vi "PipBoy_Main.vi"() -> ()   [LabVIEW 2014]
uses:
  ctls/PipBoy_LabVIEWEvent.ctl
  ctls/PipBoy_DetectionType.ctl
  <vilib>/ErrorRing/Error Ring.xnode
  modules/support/Message Queue/Message Queue.lvlib
  modules/support/User Event - Stop/User Event - Stop.lvlib
panel:
  in  "Command":string="Add"
  out "PipBoy":string
  in  "Cmd":bool
  in  "Stop":bool
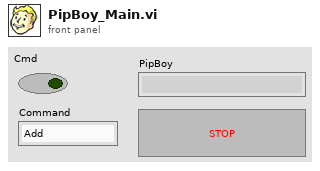
[diagram p1: front panel]
types:
  T1 = enum32{"Invalid", "Standard", "Closed", "Hidden", "Minimized", "Maximized"}
  T2 = typedef "PipBoy_PipBoyData.ctl" = cluster{"ProcComm":T3, "FileConf":T5, "PicComm":T6, "GnlPrms":T7, "Pages":T8}
  T3 = typedef "PipBoy_ProcComm.ctl" = cluster{"NotifyIconRef":refnum<k24>, "UE-Stop":refnum<user-event>, "UE-PipboyCommand":refnum<user-event>, "UE-UpdateData":refnum<user-event>, "MsgQ":T4}
  T4 = typedef "Message Queue.lvlib/All Message Queues.ctl" = cluster{"UI":refnum<queue>, "PipCom":refnum<queue>}
  T5 = typedef "PipBoy_FileConf.ctl" = cluster{"VisaPic32":refnum<visa-resource-name>, "LabVIEWPorts":u16[], "DEBUG":bool, "IconFilePath":path, "IconsNbByPage":i32}
  T6 = typedef "PipBoy_PicComm.ctl" = cluster{"PicInit?":bool}
  T7 = typedef "PipBoy_GeneralParams.ctl" = cluster{"IconPath":path, "LabVIEWs":refnum<vi>[], "ActiveLabVIEW":i32, "OpenedPorts":u16[], "ContextMenu":string[][]}
  T8 = typedef "PipBoy_Pages.ctl" = cluster{"PageNum":i32, "Functions":string[]}
  T9 = cluster{"UE-Stop":refnum<event-registration>, "UE-NotifyMenu":refnum<event-registration>, "UE-PipBoyCmd":refnum<event-registration>, "UE-UpdateData":refnum<event-registration>}
  T10 = typedef "PipBoy_LabVIEWEvent.ctl" = cluster{"DetecType":T11, "LvVersion":string, "Index":i32}
  T11 = typedef "PipBoy_DetectionType.ctl" = enum16{"Detected", "Lost"}
  T12 = typedef "NotifyIcon Event Data.ctl" = cluster{"NotifyIcon Event":T13, "Data String":string}
  T13 = typedef "NotifyIcon Events.ctl" = enum16{"BalloonTipClicked", "BalloonTipClosed", "BalloonTipShown", "Click", "Disposed", "DoubleClick", "MouseClick", "MouseDoubleClick", "MouseDown", "MouseMove", "MouseUp", "MenuItemClick", "MenuItemSelect"}
  T14 = enum32{"invalid app kind", "Development System", "Run Time System", "Student Edition", "Embedded LabVIEW", "Evaluation", "Custom"}
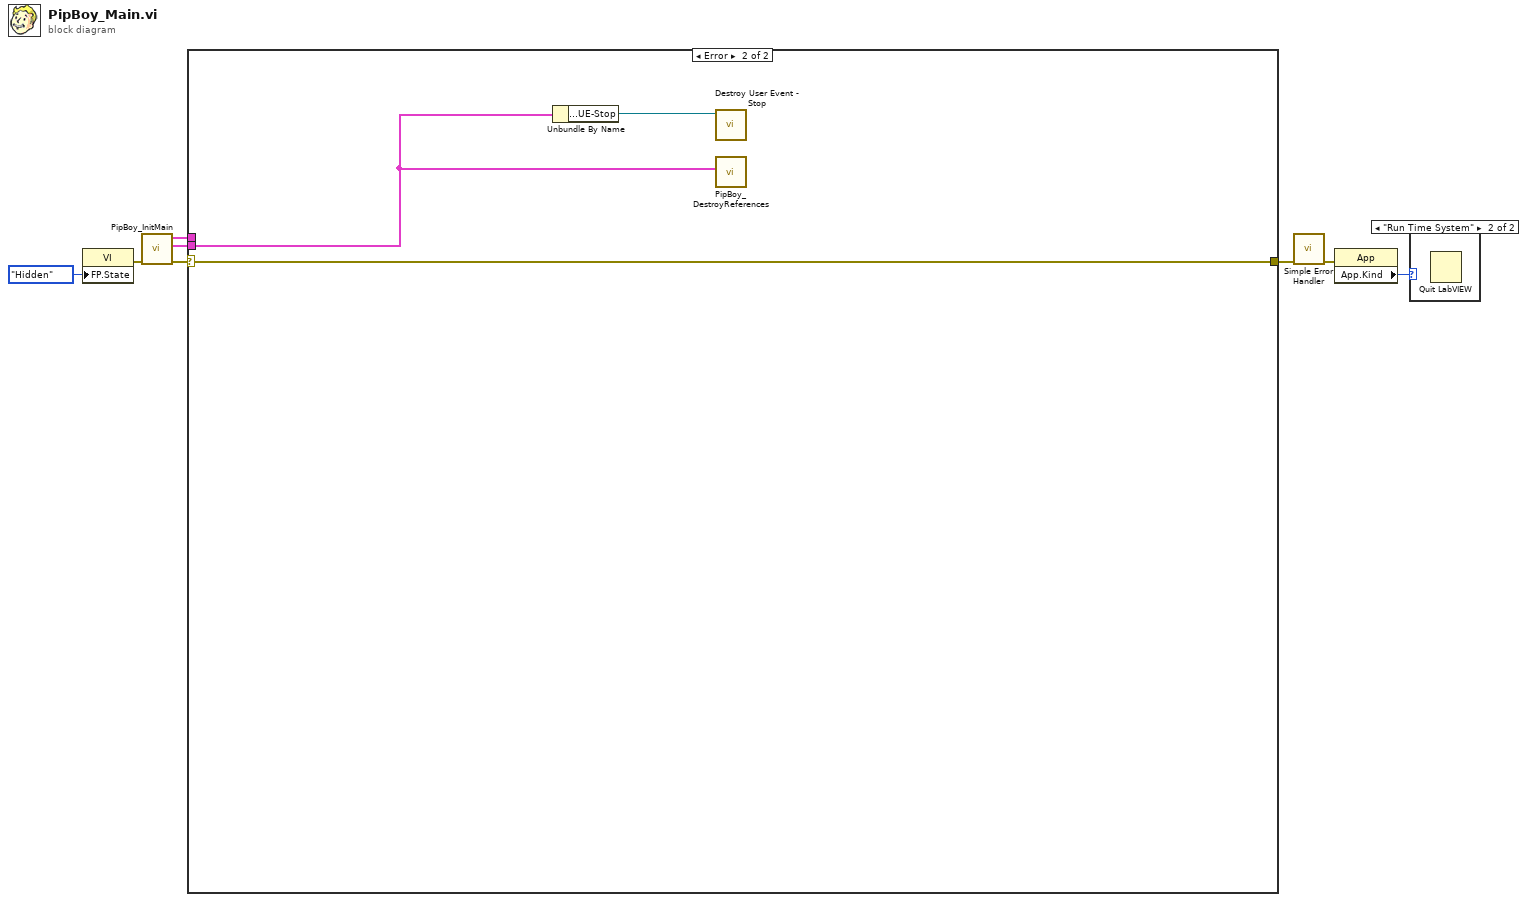
[diagram p0: block diagram]
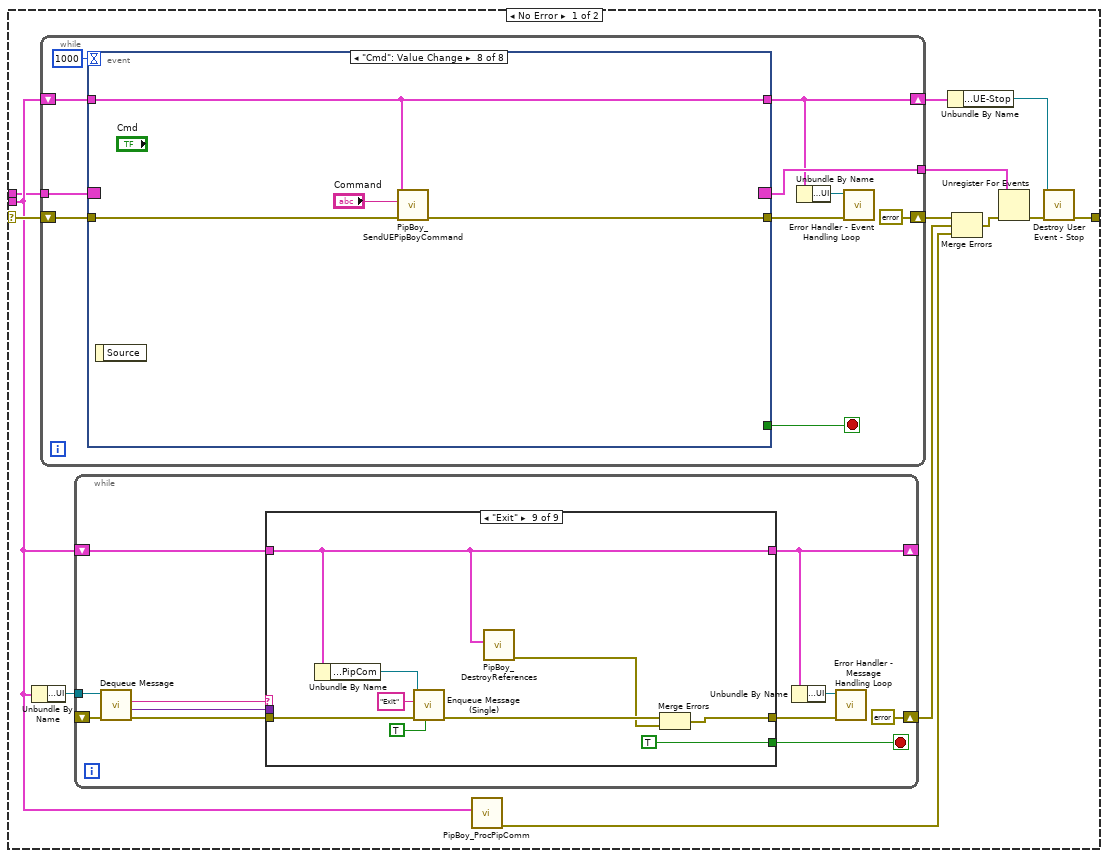
[diagram p2: hidden frame]
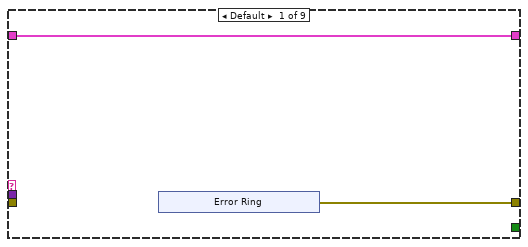
[diagram p3: hidden frame]
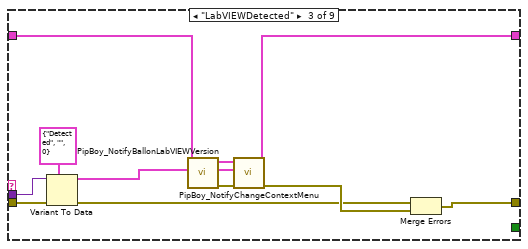
[diagram p5: hidden frame]
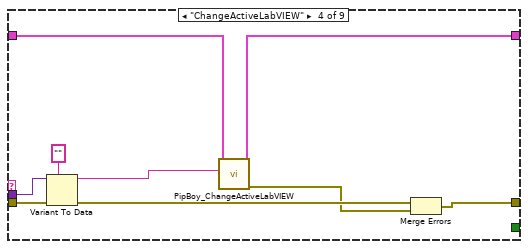
[diagram p6: hidden frame]
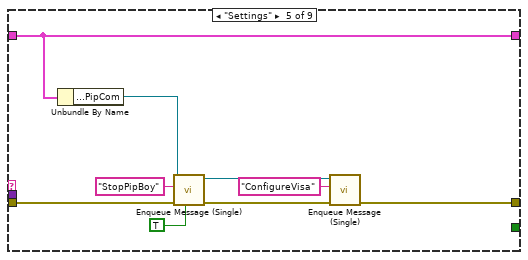
[diagram p7: hidden frame]
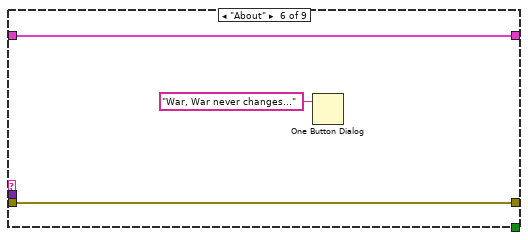
[diagram p8: hidden frame]
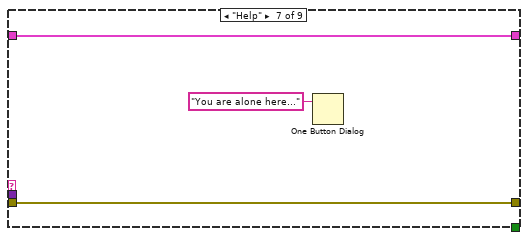
[diagram p9: hidden frame]
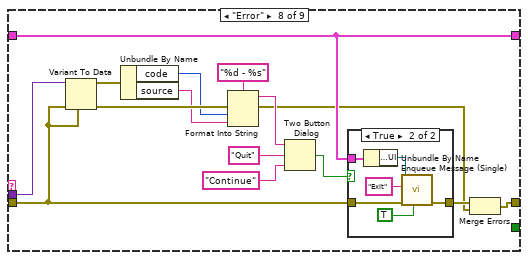
[diagram p10: hidden frame]
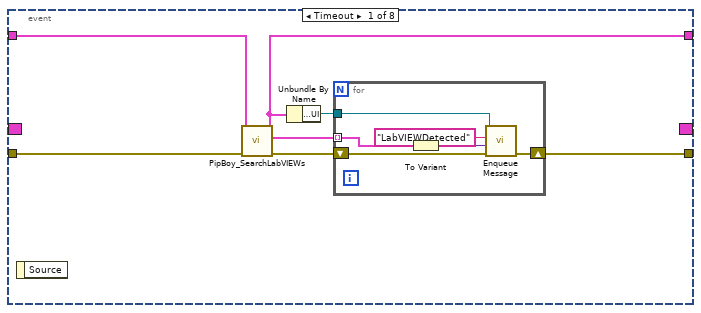
[diagram p12: hidden frame]
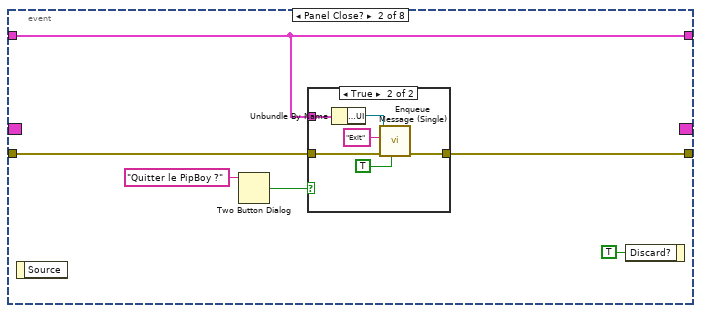
[diagram p13: hidden frame]
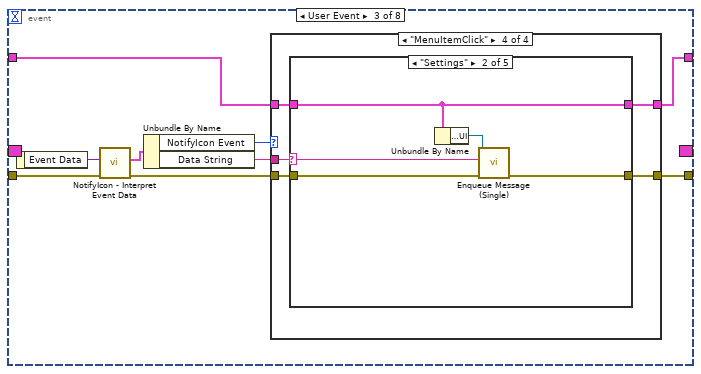
[diagram p15: hidden frame]
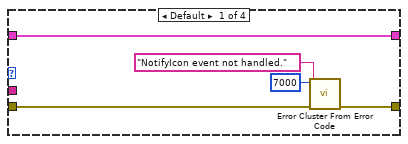
[diagram p16: hidden frame]
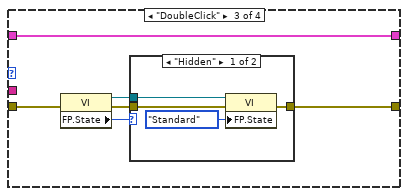
[diagram p18: hidden frame]
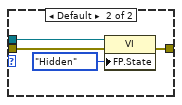
[diagram p19: hidden frame]
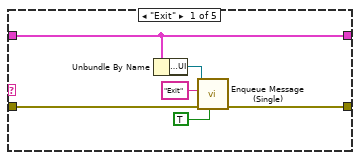
[diagram p20: hidden frame]
diagram:
  n1 = property class="VI"("FP.State"=T1."Hidden" ("Front Panel Window:State")) -> (error out=w3:errorcluster)  [unwired: 2 in, 1 out]
  n2 = call "PipBoy_InitMain.vi"("error in (no error)"=w3) -> ("error out"=w5:errorcluster, "PipBoyData"=w6:T2, "DynamicUE"=w1:T9)  [unwired: 8 in]
  n3 = case shown="Error" w5 {
    selector: w5 -> [w11 w286]
    tunnel: [w16 w286] -> w7
    tunnel: w6 -> [w10 w285]
    tunnel: w1 -> [w9 _]
    frame No Error {
      n4 = Unbundle By Name(w10) -> ("ProcComm.MsgQ.UI"=w18:refnum<queue>)
      n5 = while {
        tunnel: [w115] -> w19
        shift-right: [w112] -> w13
        shift-left: w10 -> [w113]
        shift-right: [errorcluster {"status"=FALSE, "code"=0, "source"=""} ("error IO")] -> w21
        shift-left: w11 -> [w118]
        tunnel: w9 -> [w109]
        stop <- w117 stop-if-true
        n6 = event shown="[7] \"Cmd\": Value Change" {
          selector: w109 -> [_ _ _ _ _ _ _ _]
          dyn-events: [_ _ _ _ _ _ _ _] -> w115
          timeout: 1000 -> [_ _ _ _ _ _ _ _]
          tunnel: w118 -> [w125 w135 w153 w230 w243 w264 w279 w282]
          tunnel: [_ _ _ TRUE ("Discard?") _ _ _ _] -> w117
          tunnel: [w122 w134 w148 w230 w242 w263 w276 w281] -> w116
          tunnel: w113 -> [w124 w132 w146 w229 w234 w260 w275 w283]
          tunnel: [w119 w132 w145 w229 w233 w259 w275 w283] -> w112
          event Timeout {
            n7 = event-data() -> ()  [unwired: 1 in, 1 out]
            n8 = call "PipBoy_SearchLabVIEWs.vi"("error in (no error)"=w125, "PipBoyDataIn"=w124) -> ("error out"=w123:errorcluster, "LabVIEWEvents"=w120:T10[], "PipBoyDataOut"=w119:T2)  [unwired: 7 in]
            n9 = Unbundle By Name(w119) -> ("ProcComm.MsgQ.UI"=w121:refnum<queue>)
            n10 = for {
              shift-right: [w129] -> w122
              shift-left: w123 -> [w130]
              tunnel: w121 -> [w126]
              tunnel: w120 -> [w128] mode=indexing
              n11 = To Variant(anything=w128) -> (Variant=w127:variant)
              n12 = call-poly "Enqueue Message.vi"("error in (no error)"=w130, "Message Data"=w127, "Message"="LabVIEWDetected", "Message Queue"=w126) -> ("error out"=w129:errorcluster)  [unwired: 6 in, 1 out]
            }
          }
          event Panel Close? {
            n13 = event-data() -> ()  [unwired: 1 in, 1 out]
            n14 = Two Button Dialog(message="Quitter le PipBoy ?") -> (T button?=w133:bool)  [unwired: 2 in]
            n15 = case shown="True" w133 {
              tunnel: w135 -> [w138 w142]
              tunnel: [w138 w141] -> w134
              tunnel: w132 -> [_ w140]
              frame False {
              }
              frame True {
                n16 = Unbundle By Name(w140) -> ("ProcComm.MsgQ.UI"=w139:refnum<queue>)
                n17 = call "Enqueue Message (Single).vi"("Priority Message? (F)"=TRUE, "error in (no error)"=w142, "Message"="Exit", "Message Queue"=w139) -> ("error out"=w141:errorcluster)  [unwired: 6 in, 1 out]
              }
            }
            n18 = event-data("Discard?"=TRUE) -> ()  [unwired: 1 in, 1 out]
          }
          event User Event {
            n19 = event-data() -> ("Event Data"=w152:variant)  [unwired: 1 in]
            n20 = call <userlib>:"NotifyIcon - Interpret Event Data.vi"("error in"=w153, "NotifyIcon Event Data"=w152) -> ("error out"=w149:errorcluster, "NotifyIcon Event Data"=w151:T12)  [unwired: 8 in]
            n21 = Unbundle By Name(w151) -> ("NotifyIcon Event"=w150:T13, "Data String"=w147:string)
            n22 = case shown="\"MenuItemClick\"" w150 {
              tunnel: w149 -> [w157 w160 w164 w178]
              tunnel: [w158 w160 w162 w177] -> w148
              tunnel: w147 -> [_ _ _ w179]
              tunnel: w146 -> [w154 w159 w161 w176]
              tunnel: [w154 w159 w161 w175] -> w145
              frame Default {
                n23 = call <vilib>:"Error Cluster From Error Code.vi"("error in (no error)"=w157, "error message (\"\")"="NotifyIcon event not handled." ("error message (\"\")"), "error code (0)"=7000) -> ("error out"=w158:errorcluster)  [unwired: 6 in]
              }
              frame "BalloonTipClicked" {
              }
              frame "DoubleClick" {
                n24 = property class="VI"(error in=w164) -> (reference out=w165:refnum<vi>, error out=w163:errorcluster, "FP.State"=w166:T1)  [unwired: 1 in]
                n25 = case shown="\"Hidden\"" w166 {
                  tunnel: w165 -> [w168 w171]
                  tunnel: w163 -> [w170 w173]
                  tunnel: [w169 w172] -> w162
                  frame "Hidden" {
                    n26 = property class="VI"(reference=w168, error in=w170, "FP.State"=T1."Standard" ("Front Panel Window:State")) -> (error out=w169:errorcluster)  [unwired: 1 out]
                  }
                  frame Default {
                    n27 = property class="VI"(reference=w171, error in=w173, "FP.State"=T1."Hidden" ("Front Panel Window:State")) -> (error out=w172:errorcluster)  [unwired: 1 out]
                  }
                }
              }
              frame "MenuItemClick" {
                n28 = case shown="\"Settings\"" w179 {
                  selector: w179 -> [_ w187 w192 w197 w213]
                  tunnel: w178 -> [w183 w189 w194 w199 w204]
                  tunnel: [w182 w188 w193 w198 w203] -> w177
                  tunnel: w176 -> [w180 w186 w191 w196 w202]
                  tunnel: [w180 w186 w191 w196 w201] -> w175
                  frame "Exit" {
                    n29 = Unbundle By Name(w180) -> ("ProcComm.MsgQ.UI"=w181:refnum<queue>)
                    n30 = call "Enqueue Message (Single).vi"("Priority Message? (F)"=TRUE, "error in (no error)"=w183, "Message"="Exit", "Message Queue"=w181) -> ("error out"=w182:errorcluster)  [unwired: 6 in, 1 out]
                  }
                  frame "Settings" {
                    n31 = Unbundle By Name(w186) -> ("ProcComm.MsgQ.UI"=w190:refnum<queue>)
                    n32 = call "Enqueue Message (Single).vi"("error in (no error)"=w189, "Message"=w187, "Message Queue"=w190) -> ("error out"=w188:errorcluster)  [unwired: 7 in, 1 out]
                  }
                  frame "About" {
                    n33 = Unbundle By Name(w191) -> ("ProcComm.MsgQ.UI"=w195:refnum<queue>)
                    n34 = call "Enqueue Message (Single).vi"("error in (no error)"=w194, "Message"=w192, "Message Queue"=w195) -> ("error out"=w193:errorcluster)  [unwired: 7 in, 1 out]
                  }
                  frame "Help" {
                    n35 = Unbundle By Name(w196) -> ("ProcComm.MsgQ.UI"=w200:refnum<queue>)
                    n36 = call "Enqueue Message (Single).vi"("error in (no error)"=w199, "Message"=w197, "Message Queue"=w200) -> ("error out"=w198:errorcluster)  [unwired: 7 in, 1 out]
                  }
                  frame Default {
                    n37 = Spreadsheet String To Array(delimiter (Tab)="\\", format string="", spreadsheet string=w213, array type (2D Dbl)=string[] []) -> (array=w211:string[])
                    n38 = Index Array(array=w211) -> (element #1=w209:string, element #2=w208:string)  [unwired: 2 in]
                    n39 = case shown="\"Active LabVIEW\"" w209 {
                      tunnel: w208 -> [_ w221 w224]
                      tunnel: "A town has been desolated..." -> [_ w219 _]
                      tunnel: "Barraux has been desolated..." -> [_ w218 _]
                      tunnel: w204 -> [w214 w216 w228]
                      tunnel: [w214 w216 w227] -> w203
                      tunnel: w202 -> [w215 w217 w226]
                      tunnel: [w215 w217 w225] -> w201
                      frame Default {
                      }
                      frame "Nuclear Strike" {
                        n40 = case shown="\"Random city\"" w221 {
                          tunnel: [w222 w223] -> w220
                          tunnel: w219 -> [w222 _]
                          tunnel: w218 -> [_ w223]
                          frame Default {
                          }
                          frame "Random city" {
                          }
                        }
                        n41 = One Button Dialog(message=w220) -> ()  [unwired: 1 in, 1 out]
                      }
                      frame "Active LabVIEW" {
                        n42 = call "PipBoy_ChangeActiveLabVIEW.vi"("error in (no error)"=w228, "LvVersion"=w224, "PipBoyDataIn"=w226) -> ("error out"=w227:errorcluster, "PipBoyDataOut"=w225:T2)  [unwired: 7 in]
                      }
                    }
                  }
                }
              }
            }
          }
          event User Event {
            n43 = event-data() -> ()  [unwired: 1 in, 1 out]
          }
          event User Event {
            n44 = event-data() -> ("Name"=w232:string)  [unwired: 1 in]
            "PipBoy" <- w232
            n45 = Spreadsheet String To Array(delimiter (Tab)="=", format string="", spreadsheet string=w232, array type (2D Dbl)=string[] []) -> (array=w238:string[])
            n46 = Index Array(array=w238) -> (element #1=w237:string, element #2=w236:string)  [unwired: 2 in]
            n47 = case shown="\"Icon\"" w237 {
              tunnel: [w246 w250 w253 w257] -> w242
              tunnel: w234 -> [w245 w247 w252 w256]
              tunnel: w243 -> [w246 w249 w254 w258]
              tunnel: w236 -> [_ w248 _ _]
              tunnel: [w245 w247 w251 w255] -> w233
              frame Default {
              }
              frame "Icon" {
                n48 = call "PipBoy_SendCommandToLabVIEW.vi"("error in (no error)"=w249, "Command"=w248, "PipBoyDataIn"=w247) -> ("error out"=w250:errorcluster)  [unwired: 8 in]
              }
              frame "Previous" {
                n49 = call "PipBoy_Cmd-Previous.vi"("error in (no error)"=w254, "DataIn"=w252) -> ("error out"=w253:errorcluster, "DataOut"=w251:T2)  [unwired: 8 in]
              }
              frame "Next" {
                n50 = call "PipBoy_Cmd-Next.vi"("error in (no error)"=w258, "DataIn"=w256) -> ("error out"=w257:errorcluster, "DataOut"=w255:T2)  [unwired: 8 in]
              }
            }
            n51 = Unbundle By Name(w234) -> ("FileConf.DEBUG"=w241:bool)
            n52 = case shown="True" w241 {
              tunnel: w232 -> [_ w244]
              frame False {
              }
              frame True {
                n53 = One Button Dialog(message=w244) -> ()  [unwired: 1 in, 1 out]
              }
            }
          }
          event User Event {
            n54 = event-data() -> ("Name"=w262:string, "Data"=w261:variant)  [unwired: 1 in]
            n55 = case shown="\"ContextMenu\"" w262 {
              tunnel: [w266 w270] -> w263
              tunnel: w264 -> [w266 w271]
              tunnel: w261 -> [_ w269]
              tunnel: [w265 w272] -> w259
              tunnel: w260 -> [w265 w273]
              frame Default {
              }
              frame "ContextMenu" {
                n56 = Variant To Data(error in=w271, type=string[][] [] ("GnlPrms.ContextMenu"), Variant=w269) -> (data=w267:string[][], error out=w270:errorcluster)
                n57 = Bundle By Name(cluster=w273, "GnlPrms.ContextMenu"=w267) -> (w272:T2)
              }
            }
          }
          event "Stop": Value Change {
            n58 = event-data() -> ()  [unwired: 1 in, 1 out]
            n59 = Unbundle By Name(w275) -> ("ProcComm.MsgQ.UI"=w274:refnum<queue>)
            n60 = call "Enqueue Message (Single).vi"("Priority Message? (F)"=TRUE, "error in (no error)"=w279, "Message"="Exit", "Message Queue"=w274) -> ("error out"=w276:errorcluster)  [unwired: 6 in, 1 out]
          }
          event "Cmd": Value Change {
            n61 = event-data() -> ()  [unwired: 1 in, 1 out]
            n62 = call "PipBoy_SendUEPipBoyCommand.vi"("error in (no error)"=w282, "Command"="Command", "PipBoyData"=w283) -> ("error out"=w281:errorcluster)  [unwired: 8 in]
          }
        }
        n63 = Unbundle By Name(w112) -> ("ProcComm.MsgQ.UI"=w114:refnum<queue>)
        n64 = call "Error Handler - Event Handling Loop.vi"("error in (no error)"=w116, "Message Queue"=w114) -> ()  [unwired: 8 in, 2 out]
      }
      n65 = while {
        tunnel: w18 -> [w24]
        shift-right: [errorcluster {"status"=FALSE, "code"=0, "source"=""} ("error IO")] -> w14
        shift-left: _ -> [w32]
        shift-right: [w25] -> _
        shift-left: w10 -> [w28]
        stop <- w27 stop-if-true
        n66 = call "Dequeue Message.vi"("error in (no error)"=w32, "Message Queue"=w24) -> ("error out"=w29:errorcluster, "Message Data"=w26:variant, "Message"=w31:string)  [unwired: 6 in, 1 out]
        n67 = case shown="\"Exit\"" w31 {
          tunnel: [w34 w40 w53 w62 w63 w73 w76 w83 w108] -> w30
          tunnel: w29 -> [_ w40 w47 w61 w70 w73 w76 w80 w104]
          tunnel: w28 -> [w33 w41 w52 w58 w69 w74 w77 w84 w100]
          tunnel: [w33 w41 w48 w57 w69 w74 w77 w84 w100] -> w25
          tunnel: [_ _ _ _ _ _ _ _ TRUE] -> w27
          tunnel: w26 -> [_ _ w44 w59 _ _ _ w92 _]
          frame Default {
            n68 = xnode "Error Ring"() -> ("error out"=w34:errorcluster)
          }
          frame "Initialize" {
          }
          frame "LabVIEWDetected" {
            n69 = Variant To Data(error in=w47, type=T10 {"DetecType"=enum."Detected", "LvVersion"="", "Index"=0} ("LabVIEWEvent"), Variant=w44) -> (data=w43:T10, error out=w46:errorcluster)
            n70 = call "PipBoy_NotifyBallonLabVIEWVersion.vi"("LabVIEWEventIn"=w43, "PipBoyDataIn"=w52) -> ("error out"=w51:errorcluster, "LabVIEWEventOut"=w42:T10, "PipBoyDataOut"=w49:T2)  [unwired: 7 in]
            n71 = call "PipBoy_NotifyChangeContextMenu.vi"("error in (no error)"=w51, "LabVIEWEvent"=w42, "PipBoyDataIn"=w49) -> ("error out"=w50:errorcluster, "PipBoyDataOut"=w48:T2)  [unwired: 7 in]
            n72 = Merge Errors(w46, w50) -> (w53:errorcluster)
          }
          frame "ChangeActiveLabVIEW" {
            n73 = Variant To Data(error in=w61, type="", Variant=w59) -> (data=w55:string, error out=w60:errorcluster)
            n74 = call "PipBoy_ChangeActiveLabVIEW.vi"("LvVersion"=w55, "PipBoyDataIn"=w58) -> ("error out"=w54:errorcluster, "PipBoyDataOut"=w57:T2)  [unwired: 8 in]
            n75 = Merge Errors(w60, w54) -> (w62:errorcluster)
          }
          frame "Settings" {
            n76 = Unbundle By Name(w69) -> ("ProcComm.MsgQ.PipCom"=w68:refnum<queue>)
            n77 = call "Enqueue Message (Single).vi"("Priority Message? (F)"=TRUE, "error in (no error)"=w70, "Message"="StopPipBoy", "Message Queue"=w68) -> ("error out"=w64:errorcluster, "dup Message Queue"=w67:refnum<queue>)  [unwired: 6 in]
            n78 = call "Enqueue Message (Single).vi"("error in (no error)"=w64, "Message"="ConfigureVisa", "Message Queue"=w67) -> ("error out"=w63:errorcluster)  [unwired: 7 in, 1 out]
          }
          frame "About" {
            n79 = One Button Dialog(message="War, War never changes...") -> ()  [unwired: 1 in, 1 out]
          }
          frame "Help" {
            n80 = One Button Dialog(message="You are alone here...") -> ()  [unwired: 1 in, 1 out]
          }
          frame "Error" {
            n81 = Variant To Data(error in=w80, type=w80, Variant=w92) -> (data=w91:errorcluster, error out=w90:errorcluster)
            n82 = Unbundle By Name(w91) -> ("code"=w89:i32, "source"=w87:string)
            n83 = Format Into String(format string="%d - %s", error in=w90, w89, w87) -> (resulting string=w86:string, error out=w81:errorcluster)  [unwired: 1 in]
            n84 = Two Button Dialog(message=w86, 1:"Continue" ("F button name (\"Cancel\")"), 2:"Quit" ("T button name (\"OK\")")) -> (T button?=w85:bool)
            n85 = case shown="True" w85 {
              tunnel: [w93 w97] -> w82
              tunnel: w80 -> [w93 w96]
              tunnel: w84 -> [_ w95]
              frame False {
              }
              frame True {
                n86 = Unbundle By Name(w95) -> ("ProcComm.MsgQ.UI"=w94:refnum<queue>)
                n87 = call "Enqueue Message (Single).vi"("Priority Message? (F)"=TRUE, "error in (no error)"=w96, "Message"="Exit", "Message Queue"=w94) -> ("error out"=w97:errorcluster)  [unwired: 6 in, 1 out]
              }
            }
            n88 = Merge Errors(w82, w81) -> (w83:errorcluster)
          }
          frame "Exit" {
            n89 = Unbundle By Name(w100) -> ("ProcComm.MsgQ.PipCom"=w103:refnum<queue>)
            n90 = call "Enqueue Message (Single).vi"("Priority Message? (F)"=TRUE, "error in (no error)"=w104, "Message"="Exit", "Message Queue"=w103) -> ("error out"=w102:errorcluster)  [unwired: 6 in, 1 out]
            n91 = call "PipBoy_DestroyReferences.vi"("PipBoyData"=w100) -> ("error out"=w101:errorcluster)  [unwired: 10 in]
            n92 = Merge Errors(w102, w101) -> (w108:errorcluster)
          }
        }
        n93 = Unbundle By Name(w25) -> ("ProcComm.MsgQ.UI"=w23:refnum<queue>)
        n94 = call "Error Handler - Message Handling Loop.vi"("error in (no error)"=w30, "Message Queue"=w23) -> ()  [unwired: 8 in, 2 out]
      }
      n95 = call "PipBoy_ProcPipComm.vi"("PipBoyData"=w10) -> ("error out"=w12:errorcluster)  [unwired: 10 in]
      n96 = Unbundle By Name(w13) -> ("ProcComm.UE-Stop"=w15:refnum<user-event>)
      n97 = Merge Errors(w21, w14, w12) -> (w20:errorcluster)
      n98 = Unregister For Events(event registration refnum=w19, error in=w20) -> (error out=w17:errorcluster)
      n99 = call "Destroy User Event - Stop.vi"("error in (no error)"=w17, "User Event - Stop"=w15) -> ("error out"=w16:errorcluster)  [unwired: 9 in]
    }
    frame Error {
      n100 = Unbundle By Name(w285) -> ("ProcComm.UE-Stop"=w284:refnum<user-event>)
      n101 = call "Destroy User Event - Stop.vi"("User Event - Stop"=w284) -> ()  [unwired: 10 in, 1 out]
      n102 = call "PipBoy_DestroyReferences.vi"("PipBoyData"=w285) -> ()  [unwired: 10 in, 1 out]
    }
  }
  n103 = call <vilib>:"Simple Error Handler.vi"("error in (no error)"=w7) -> ("error out"=w8:errorcluster)  [unwired: 4 in, 4 out]
  n104 = property class="App"(error in=w8) -> ("App.Kind"=w4:T14)  [unwired: 1 in, 2 out]
  n105 = case shown="\"Run Time System\"" w4 {
    frame "invalid app kind", Default {
    }
    frame "Run Time System" {
      n106 = Quit LabVIEW() -> ()  [unwired: 1 in]
    }
  }
